vi "OutputRF.vi"(6 "Cal Routes":string[](array[string]), 7 "output enabled":bool=TRUE, 8 "error in (no error)":errorcluster, 9 "Power (dBm)":dbl, 10 "Frequency (Hz)":dbl, 11 "SigGen_NIRF in":refnum<class "SigGen_NIRF.lvclass">) -> (0 "error out":errorcluster, 3 "SigGen_NIRF out":refnum<class "SigGen_NIRF.lvclass">)   [LabVIEW 2014, in "SigGen_NIRF.lvclass"]
uses:
  SigGen_NIRF.lvclass
  SigGen_NIRF.lvclass/SigGen_NIRF.ctl
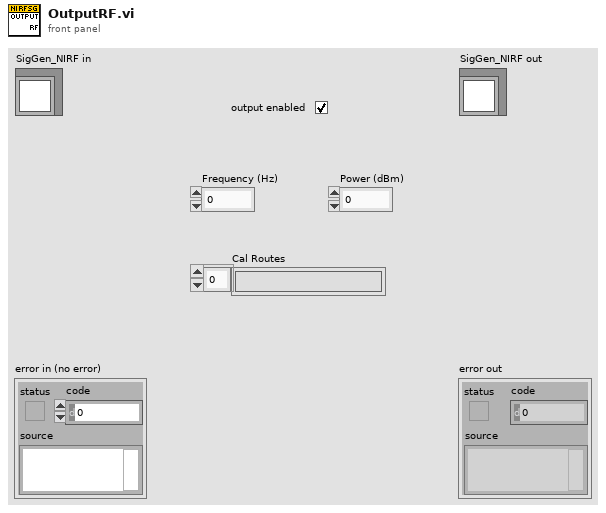
[diagram p1: front panel]
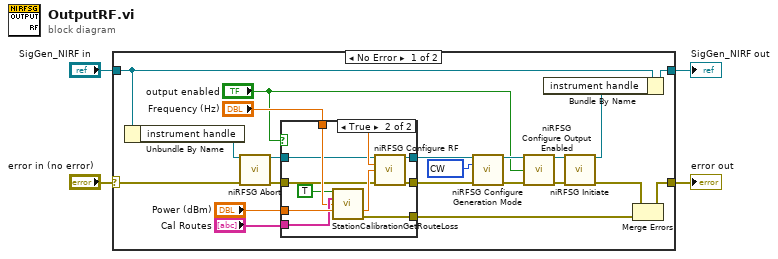
[diagram p0: block diagram]
diagram:
  n1 = case shown="No Error" "error in (no error)" {
    selector: "error in (no error)" -> [w8 w38]
    tunnel: "SigGen_NIRF in" -> [w13 w39]
    tunnel: [w19 w38] -> w2
    tunnel: [w12 w39] -> w1
    frame No Error {
      w25 = 1000 items=["CW"=1000, "Arb Waveform"=1001, "Script"=1002] ("generation mode")
      n2 = Unbundle By Name(w13) -> ("instrument handle"=w6:refnum<k15>)
      n3 = call "niRFSG Abort.vi"("instrument handle"=w6, "error in"=w8) -> ("instrument handle out"=w5:refnum<k15>, "error out"=w7:errorcluster)  [unwired: 12 in]
      n4 = case shown="True" "output enabled" {
        tunnel: w5 -> [w26 w29]
        tunnel: w7 -> [w27 w28]
        tunnel: "Power (dBm)" -> [_ w37]
        tunnel: "Cal Routes" -> [_ w36]
        tunnel: "Frequency (Hz)" -> [_ w35]
        tunnel: [w27 w33] -> w18
        tunnel: [w26 w31] -> w17
        tunnel: [w27 w30] -> w16
        frame False {
        }
        frame True {
          n5 = call "StationCalibrationGetRouteLoss.vi"("Calibration Enabled"=TRUE, "Route Names"=w36, "Frequency"=w35, "Power Level"=w37) -> ("Adjusted Power Level"=w34:dbl, "error out"=w33:errorcluster)  [unwired: 8 in, 2 out]
          n6 = call "niRFSG Configure RF.vi"("instrument handle"=w29, "frequency (Hz)"=w35, "power level (dBm)"=w34, "error in"=w28) -> ("instrument handle out"=w31:refnum<k15>, "error out"=w30:errorcluster)  [unwired: 10 in]
        }
      }
      n7 = call "niRFSG Configure Generation Mode.vi"("instrument handle"=w17, "generation mode"=w25, "error in"=w16) -> ("instrument handle out"=w24:refnum<k15>, "error out"=w23:errorcluster)  [unwired: 11 in]
      n8 = call "niRFSG Configure Output Enabled.vi"("instrument handle"=w24, "output enabled"="output enabled", "error in"=w23) -> ("instrument handle out"=w15:refnum<k15>, "error out"=w14:errorcluster)  [unwired: 11 in]
      n9 = call "niRFSG Initiate.vi"("instrument handle"=w15, "error in"=w14) -> ("instrument handle out"=w10:refnum<k15>, "error out"=w11:errorcluster)  [unwired: 12 in]
      n10 = Bundle By Name(cluster=w13, "instrument handle"=w10) -> (w12:refnum<class "SigGen_NIRF.lvclass">)
      n11 = Merge Errors(w11, w18) -> (w19:errorcluster)
    }
    frame Error {
    }
  }
  "error out" <- w2
  "SigGen_NIRF out" <- w1
